vi "RichToFlatnixnet_grpc_FrameBufferResponse.vi"(5 "OutputClusterType":T1, 11 "InputCluster":T8) -> (3 "OutputCluster":T1)   [LabVIEW 2025, in "grpc-xnet_client.lvlib"]
uses:
  nixnet_grpc_FrameBufferResponse.ctl
  nixnet_grpc_FrameBufferResponse_frame/nixnet_grpc_FrameBufferResponse_frame.lvclass
  nixnet_grpc_FrameBufferResponse_Flat.ctl
  nixnet_grpc_FrameResponse_Flat.ctl
  nixnet_grpc_FrameType.ctl
  nixnet_grpc_FrameFlags.ctl
  nixnet_grpc_EnetFrameResponse_Flat.ctl
  nixnet_grpc_EnetFrameType.ctl
  nixnet_grpc_EnetFlags.ctl
  grpc-xnet_client.lvlib
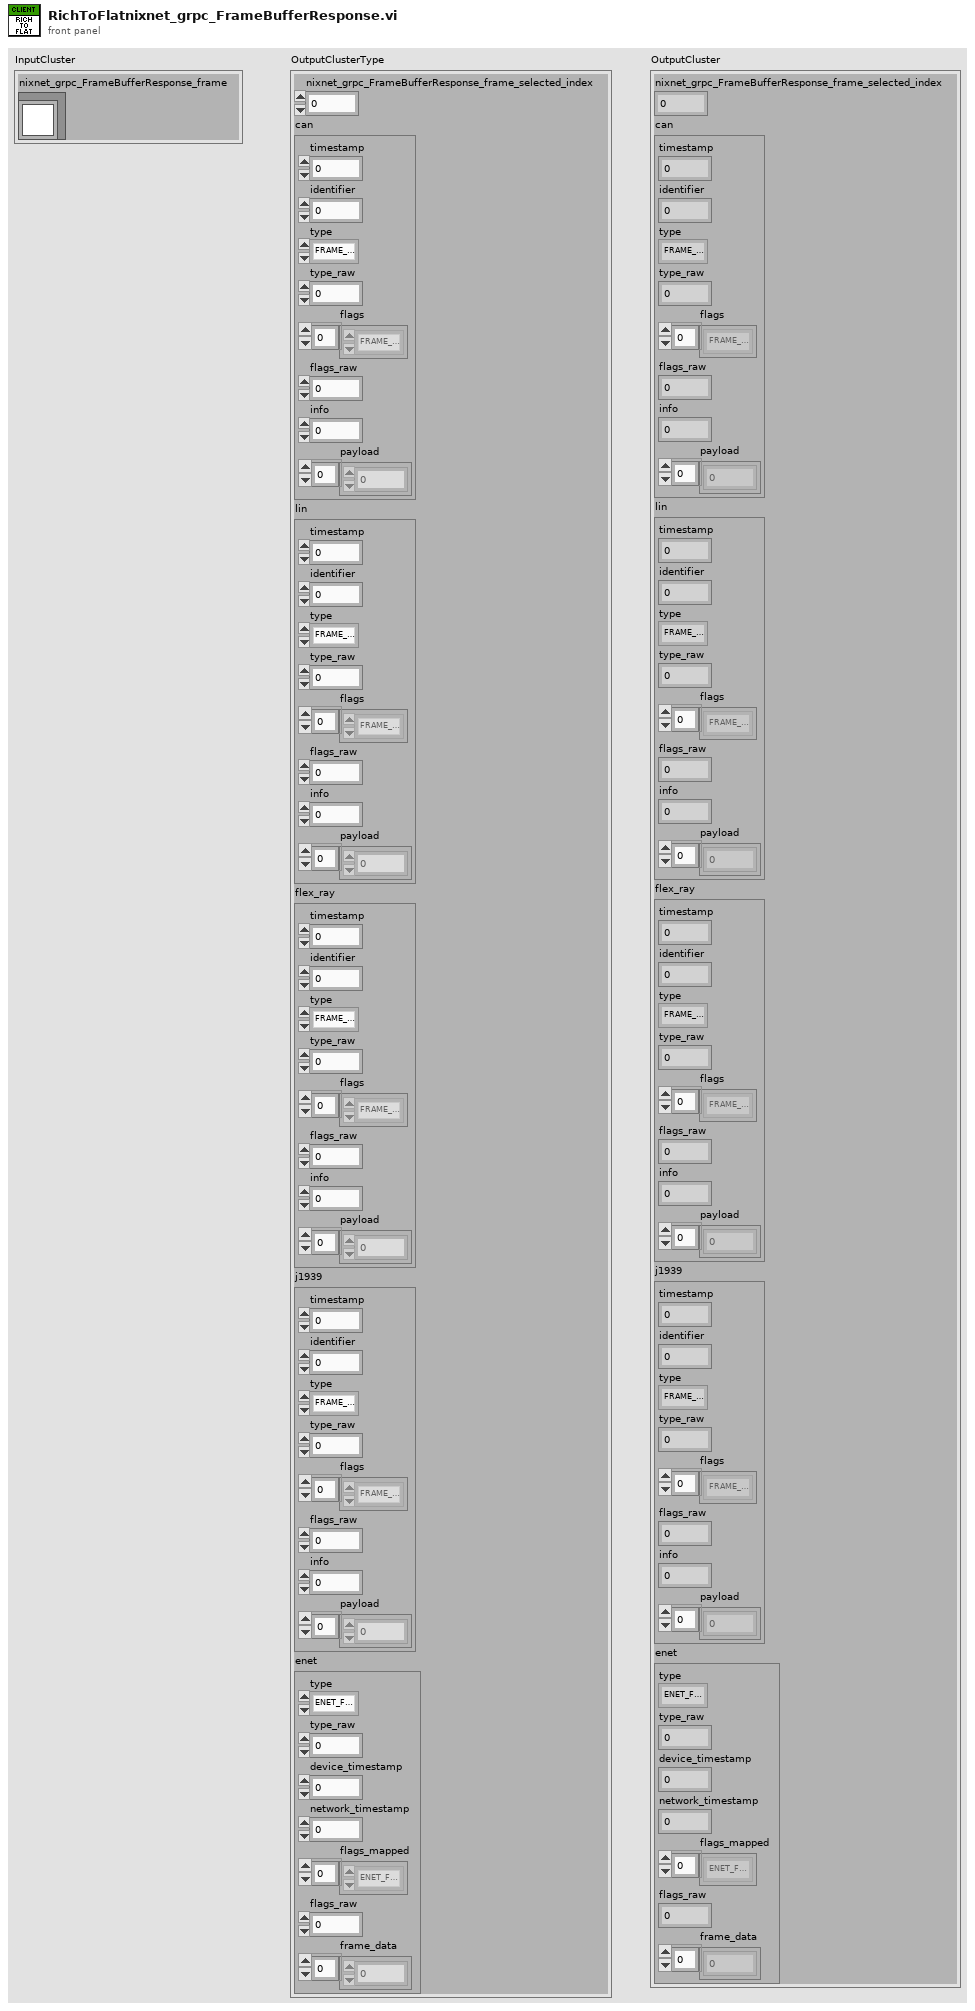
[diagram p1: front panel]
types:
  T1 = typedef "grpc-xnet_client.lvlib/nixnet_grpc_FrameBufferResponse_Flat.ctl" = cluster{"nixnet_grpc_FrameBufferResponse_frame_selected_index":i32, "can":T2, "lin":T2, "flex_ray":T2, "j1939":T2, "enet":T5}
  T2 = typedef "grpc-xnet_client.lvlib/nixnet_grpc_FrameResponse_Flat.ctl" = cluster{"timestamp":u64, "identifier":u32, "type":T3, "type_raw":u32, "flags":T4[], "flags_raw":u32, "info":u32, "payload":u8[]}
  T3 = typedef "grpc-xnet_client.lvlib/nixnet_grpc_FrameType.ctl" = enum32{"FRAME_TYPE_CAN_DATA", "FRAME_TYPE_CAN_REMOTE", "FRAME_TYPE_CAN_BUS_ERROR", "FRAME_TYPE_CAN20_DATA", "FRAME_TYPE_CANFD_DATA", "FRAME_TYPE_CANFDBRS_DATA", "FRAME_TYPE_FLEX_RAY_DATA", "FRAME_TYPE_FLEX_RAY_NULL", "FRAME_TYPE_FLEX_RAY_SYMBOL", "FRAME_TYPE_LIN_DATA", "FRAME_TYPE_LIN_BUS_ERROR", "FRAME_TYPE_LIN_NO_RESPONSE", "FRAME_TYPE_J1939_DATA", "FRAME_TYPE_SPECIAL_DELAY", "FRAME_TYPE_SPECIAL_LOG_TRIGGER", "FRAME_TYPE_SPECIAL_START_TRIGGER"}
  T4 = typedef "grpc-xnet_client.lvlib/nixnet_grpc_FrameFlags.ctl" = enum32{"FRAME_FLAGS_UNSPECIFIED", "FRAME_FLAGS_FLEX_RAY_STARTUP", "FRAME_FLAGS_FLEX_RAY_SYNC", "FRAME_FLAGS_FLEX_RAY_PREAMBLE", "FRAME_FLAGS_FLEX_RAY_CH_A", "FRAME_FLAGS_FLEX_RAY_CH_B", "FRAME_FLAGS_LIN_EVENT_SLOT", "FRAME_FLAGS_TRANSMIT_ECHO"}
  T5 = typedef "grpc-xnet_client.lvlib/nixnet_grpc_EnetFrameResponse_Flat.ctl" = cluster{"type":T6, "type_raw":u32, "device_timestamp":u64, "network_timestamp":u64, "flags_mapped":T7[], "flags_raw":u32, "frame_data":u8[]}
  T6 = typedef "grpc-xnet_client.lvlib/nixnet_grpc_EnetFrameType.ctl" = enum32{"ENET_FRAME_TYPE_DATA", "ENET_FRAME_TYPE_DELAY", "ENET_FRAME_TYPE_FUTURE_TIME_WAIT"}
  T7 = typedef "grpc-xnet_client.lvlib/nixnet_grpc_EnetFlags.ctl" = enum32{"ENET_FLAGS_UNSPECIFIED", "ENET_FLAGS_TRANSMIT", "ENET_FLAGS_RECEIVE", "ENET_FLAGS_NETWORK_SYNCED", "ENET_FLAGS_ERROR"}
  T8 = typedef "grpc-xnet_client.lvlib/nixnet_grpc_FrameBufferResponse.ctl" = cluster{"nixnet_grpc_FrameBufferResponse_frame":refnum<class "nixnet_grpc_FrameBufferResponse_frame.lvclass">}
  T9 = typedef "grpc-xnet_client.lvlib/nixnet_grpc_FrameResponse.ctl" = cluster{"timestamp":u64, "identifier":u32, "type":T3, "type_raw":u32, "flags":T4[], "flags_raw":u32, "info":u32, "payload":u8[]}
  T10 = typedef "grpc-xnet_client.lvlib/nixnet_grpc_EnetFrameResponse.ctl" = cluster{"type":T6, "type_raw":u32, "device_timestamp":u64, "network_timestamp":u64, "flags_mapped":T7[], "flags_raw":u32, "frame_data":u8[]}
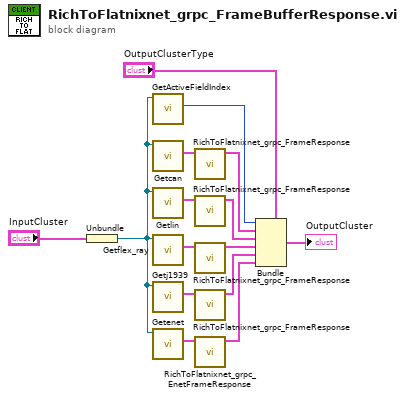
[diagram p0: block diagram]
diagram:
  n1 = Unbundle "Unbundle"("InputCluster") -> ("nixnet_grpc_FrameBufferResponse_frame"=w12:refnum<class "nixnet_grpc_FrameBufferResponse_frame.lvclass">)
  n2 = call "GetActiveFieldIndex.vi"("OneOfTemplate in"=w12) -> ("Active Field Index"=w11:i32)  [unwired: 8 in, 2 out]
  n3 = call "Getcan.vi"("OneOfTemplate in"=w12) -> ("Get_Val"=w10:T9)  [unwired: 8 in, 2 out]
  n4 = call "Getlin.vi"("OneOfTemplate in"=w12) -> ("Get_Val"=w8:T9)  [unwired: 8 in, 2 out]
  n5 = call "Getflex_ray.vi"("OneOfTemplate in"=w12) -> ("Get_Val"=w6:T9)  [unwired: 8 in, 2 out]
  n6 = call "Getj1939.vi"("OneOfTemplate in"=w12) -> ("Get_Val"=w4:T9)  [unwired: 8 in, 2 out]
  n7 = call "Getenet.vi"("OneOfTemplate in"=w12) -> ("Get_Val"=w2:T10)  [unwired: 8 in, 2 out]
  n8 = call "RichToFlatnixnet_grpc_FrameResponse.vi"("InputCluster"=w10) -> ("OutputCluster"=w9:T2)  [unwired: 10 in]
  n9 = call "RichToFlatnixnet_grpc_FrameResponse.vi"("InputCluster"=w8) -> ("OutputCluster"=w7:T2)  [unwired: 10 in]
  n10 = call "RichToFlatnixnet_grpc_FrameResponse.vi"("InputCluster"=w6) -> ("OutputCluster"=w5:T2)  [unwired: 10 in]
  n11 = call "RichToFlatnixnet_grpc_FrameResponse.vi"("InputCluster"=w4) -> ("OutputCluster"=w3:T2)  [unwired: 10 in]
  n12 = call "RichToFlatnixnet_grpc_EnetFrameResponse.vi"("InputCluster"=w2) -> ("OutputCluster"=w1:T5)  [unwired: 10 in]
  n13 = Bundle "Bundle"(cluster="OutputClusterType", "nixnet_grpc_FrameBufferResponse_frame_selected_index"=w11, "can"=w9, "lin"=w7, "flex_ray"=w5, "j1939"=w3, "enet"=w1) -> (→"OutputCluster":T1)
